vi "setCamera.vi"(8 "error in (no error)":errorcluster, 10 "Camera":enum16{"AndorIKon", "ICCamera"}(ring)=enum."ICCamera", 11 "CameraTempController.lvclass in":refnum<class "CameraTempController.lvclass">) -> (0 "error out":errorcluster, 3 "CameraTempController.lvclass out":refnum<class "CameraTempController.lvclass">)   [LabVIEW 2009, in "Hardware.lvlib" / "Channels.lvlib" / "CameraTempController.lvclass"]
uses:
  CameraTempController.lvclass
  CameraTempController.lvclass/CameraTempController.ctl
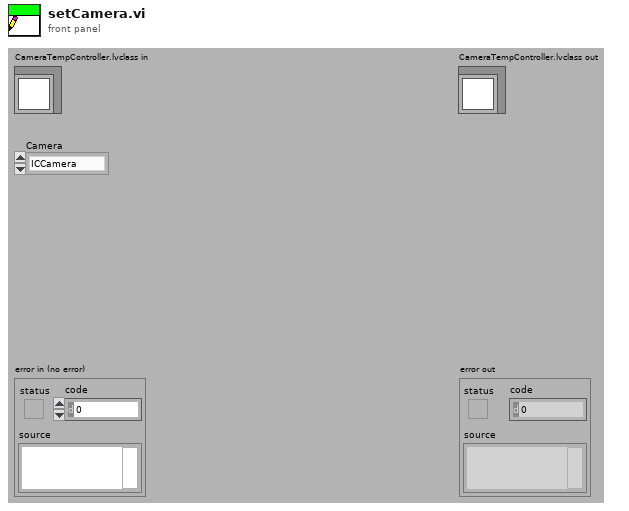
[diagram p1: front panel]
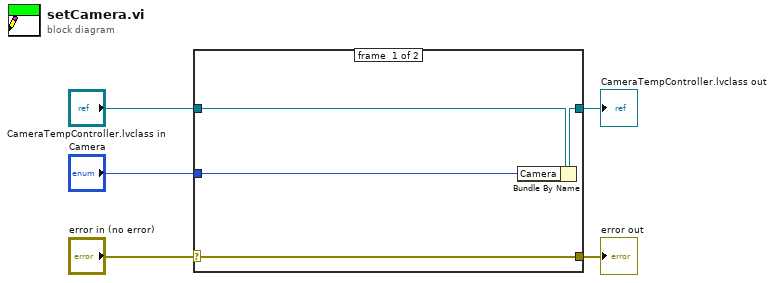
[diagram p0: block diagram]
diagram:
  n1 = case shown="No Error" "error in (no error)" {
    selector: "error in (no error)" -> [w9 w10]
    tunnel: [w9 w10] -> w4
    tunnel: [w7 w11] -> w2
    tunnel: "CameraTempController.lvclass in" -> [w8 w11]
    tunnel: "Camera" -> [w6 _]
    frame #0 {
      n2 = Bundle By Name(cluster=w8, "Camera"=w6) -> (w7:refnum<class "CameraTempController.lvclass">)
    }
    frame #1 {
    }
  }
  "error out" <- w4
  "CameraTempController.lvclass out" <- w2
